vi "FineReport_Insert.vi"(7 "InsertTableName":string, 8 "error in":errorcluster caption="error out", 9 "InsertValue(array)":string[](array[string]), 10 "InsertColumn(array)":string[](array[string]), 11 "ADODB._Connection in":refnum<k7>) -> (0 "error out":errorcluster, 3 "ADODB._Connection Out":refnum<k7>)   [LabVIEW 2018]
panel:
  # "Rev2.0"
  # "Input"
  # "Output"
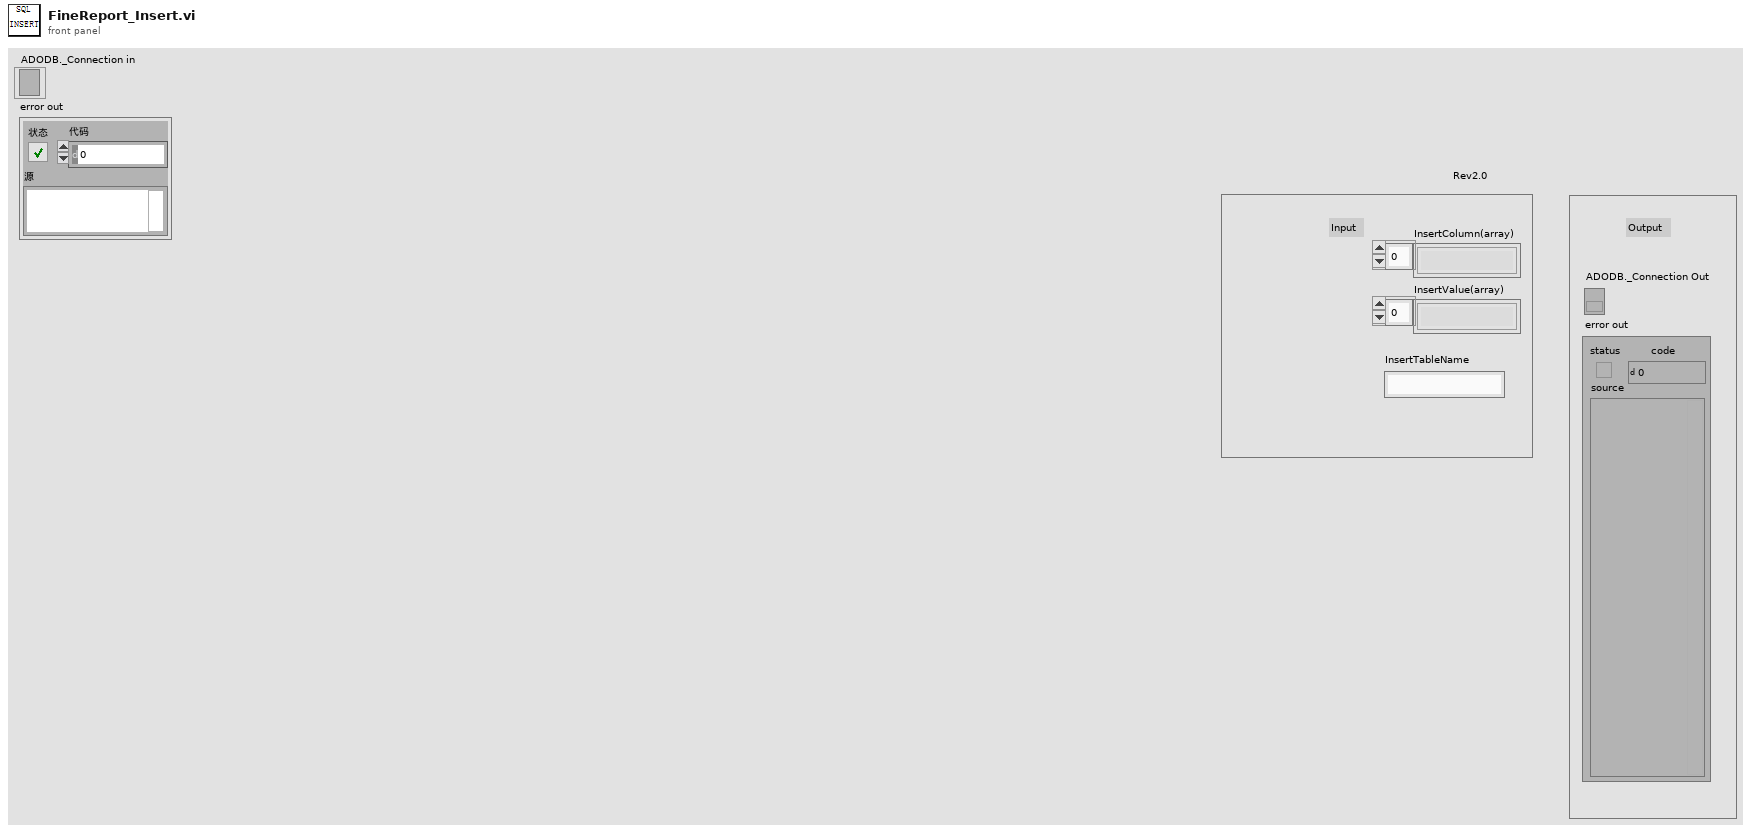
[diagram p1: front panel]
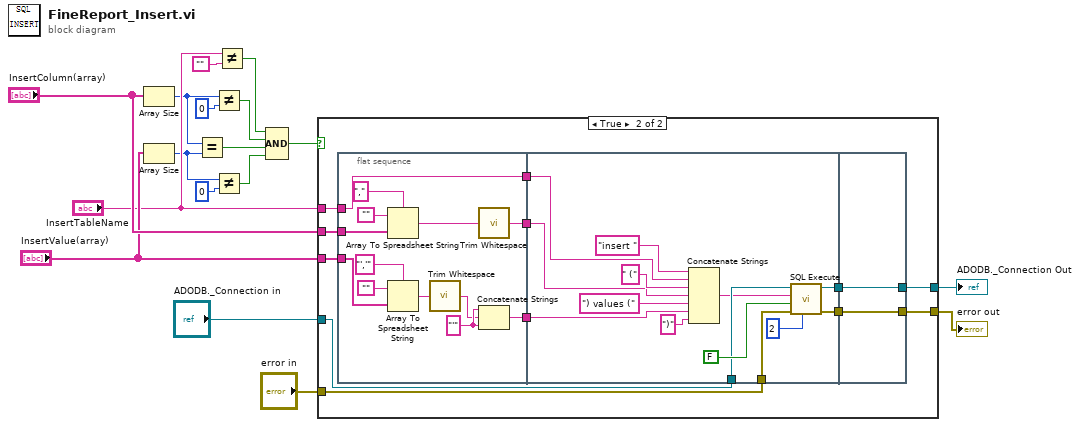
[diagram p0: block diagram]
diagram:
  n1 = Array Size(array="InsertColumn(array)") -> (size(s)=w9:i32)
  n2 = Array Size(array="InsertValue(array)") -> (size(s)=w8:i32)
  n3 = Equal?(x=w9, y=w8) -> (x = y?=w5:bool)
  n4 = Not Equal?(x=w9, y=0) -> (x != y?=w6:bool)
  n5 = Not Equal?(x=w8, y=0) -> (x != y?=w4:bool)
  n6 = Not Equal?(x="InsertTableName", y="") -> (x != y?=w7:bool)
  n7 = Compound Arithmetic op=AND(w7, w6, w5, w4) -> (w3:bool)
  n8 = case shown="True" w3 {
    tunnel: "ADODB._Connection in" -> [w19 w31]
    tunnel: "error in" -> [w18 w30]
    tunnel: [w19 w29] -> w16
    tunnel: [w18 w28] -> w15
    tunnel: "InsertColumn(array)" -> [_ w25]
    tunnel: "InsertValue(array)" -> [_ w23]
    tunnel: "InsertTableName" -> [_ w20]
    frame False {
    }
    frame True {
      n9 = flat-sequence {
        tunnel: w25 -> [w44]
        tunnel: [w34] -> w24
        tunnel: w23 -> [w39]
        tunnel: [w37] -> w22
        tunnel: [w36] -> w21
        tunnel: w20 -> [w36]
        tunnel: w31 -> [w56]
        tunnel: w30 -> [w55]
        tunnel: [w54] -> w27
        tunnel: [w46] -> w26
        tunnel: w24 -> [w51]
        tunnel: w22 -> [w50]
        tunnel: w21 -> [w49]
        tunnel: [w59] -> w28
        tunnel: [w60] -> w29
        tunnel: w27 -> [w60]
        tunnel: w26 -> [w59]
        frame #0 {
          w38 = "'" ("分隔符(Tab)")
          n10 = Array To Spreadsheet String(delimiter (Tab)="," ("分隔符(Tab)"), array=w44, 3:"" ("y")) -> (spreadsheet string=w35:string)
          n11 = Array To Spreadsheet String(delimiter (Tab)="','" ("分隔符(Tab)"), array=w39, 3:"" ("y")) -> (spreadsheet string=w33:string)
          n12 = call <vilib>:"Trim Whitespace.vi"("string"=w33) -> ("trimmed string"=w32:string)  [unwired: 1 in]
          n13 = call <vilib>:"Trim Whitespace.vi"("string"=w35) -> ("trimmed string"=w34:string)  [unwired: 1 in]
          n14 = Concatenate Strings(w38, w32, w38) -> (w37:string)
        }
        frame #1 {
          n15 = Concatenate Strings("insert ", w49, " (" ("字符串"), w51, ") values (" ("字符串"), w50, ")" ("字符串")) -> (w45:string)
          n16 = call <userlib>:"SQL Execute.vi"("Retries"=2, "error in (no error)"=w55, "Return Data (T)"=FALSE, "Command Text"=w45, "ADODB._Connection In"=w56) -> ("error out"=w46:errorcluster, "ADODB._Connection Out"=w54:refnum<k7>)  [unwired: 3 in, 2 out]
        }
        frame #2 {
        }
      }
    }
  }
  "ADODB._Connection Out" <- w16
  "error out" <- w15
